vi "CreateMenuOccurance.vi"() -> (1 "Menu Ready Occurrance":refnum<k4>, 2 "Global Menu Refnum Set":refnum<k4>)   [LabVIEW 2010]
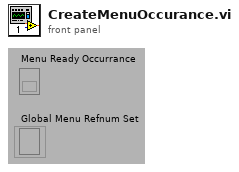
[diagram p1: front panel]
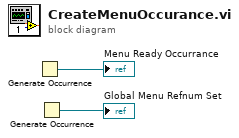
[diagram p0: block diagram]
diagram:
  n1 = Generate Occurrence() -> (→"Menu Ready Occurrance":refnum<k4>)
  n2 = Generate Occurrence() -> (→"Global Menu Refnum Set":refnum<k4>)
